vi "RSZVB Calibration Connector Catalog.vi"(8 "error in (no error)":errorcluster {"code" format="%.0x"}, 11 "VISA session":refnum<visa-resource-name>) -> (0 "error out":errorcluster {"code" format="%.0x"}, 1 "Catalog":string, 3 "dup VISA session":refnum<visa-resource-name>)   [LabVIEW 2011]
doc: "This VI returns a list of the connector types of all calibration kits in use.\n\nRemote-control command(s):\n[SENSe<Ch>:]CORRection:CONNection:CATalog?"
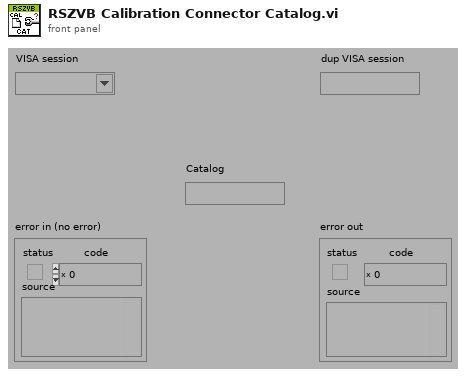
[diagram p1: front panel]
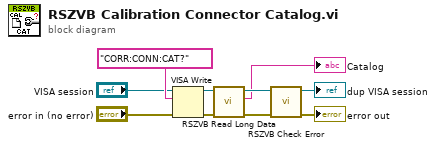
[diagram p0: block diagram]
diagram:
  n1 = VISA Write(VISA resource name="VISA session", write buffer="CORR:CONN:CAT?", error in (no error)="error in (no error)") -> (VISA resource name out=w5:refnum<visa-resource-name>, error out=w2:errorcluster)  [unwired: 1 out]
  n2 = call "RSZVB Read Long Data.vi"("error in (no error)"=w2, "VISA resource name"=w5) -> ("error out"=w3:errorcluster, "Data"=→"Catalog":string, "VISA resource name out"=w4:refnum<visa-resource-name>)  [unwired: 7 in]
  n3 = call "RSZVB Check Error.vi"("error in (no error)"=w3, "VISA session"=w4) -> ("error out"=→"error out":errorcluster, "dup VISA session"=→"dup VISA session":refnum<visa-resource-name>)  [unwired: 8 in]
